vi "mod_Apply Doppler Filter.vi"(0 "input samples":cdb[](array[numeric]), 5 "doppler filter taps":dbl[](array[numeric]), 11 "error in (no error)":errorcluster, 13 "reset (T)":bool=TRUE) -> (4 "filtered output":cdb[](array[numeric]), 15 "error out":errorcluster)   [LabVIEW 2020, in "niDMT.lvlib"]
doc: "The input signal samples are filtered out through the Doppler filter, which is a kind of low-pass filter with the cut-off frequency of the Doppler frequency and with U-shaped passband gains, although other low-pass filters have flat or equi-ripple gains.\n\n\n Inputs:\n 1) Doppler frequency (Hz) \n - range : double precision\n 2) Input samples : the input signal samples in time domain\n 3) Sampling frequency : the sampling frequency of the input samples\n 4) Filter length : the number of taps in the filter\n\n Outputs:\n 1) Filtered output : the filtered output in time domain"
uses:
  <vilib>/addons/Modulation/niDMT.lvlib
  <vilib>/Analysis/3filter.llb/IIR Filter (DBL).vi
  <vilib>/Analysis/NI_AALBase.lvlib
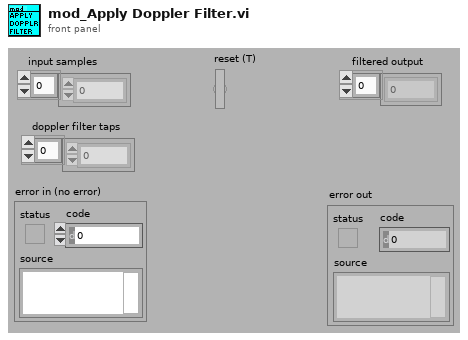
[diagram p1: front panel]
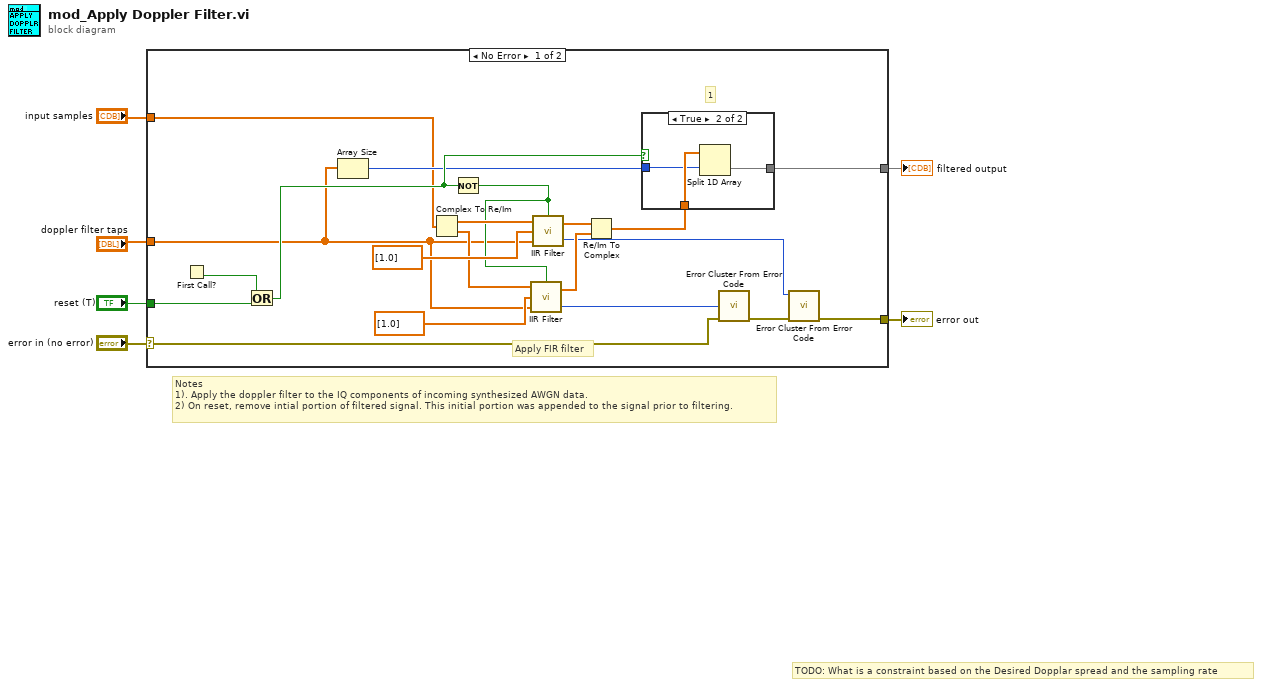
[diagram p0: block diagram]
diagram:
  # "Notes\n1). Apply the doppler filter to the IQ components of incoming synthesized AWGN data.\n2) On reset, remove intial portion of filtered signal. This initial portion was appended to the signal prior to filtering."
  # "TODO: What is a constraint based on the Desired Dopplar spread and the sampling rate"
  n1 = case shown="No Error" "error in (no error)" {
    selector: "error in (no error)" -> [w16 w31]
    tunnel: [w13 w31] -> w5
    tunnel: "input samples" -> [w10 _]
    tunnel: "doppler filter taps" -> [w9 _]
    tunnel: [w8 _] -> w2
    tunnel: "reset (T)" -> [w7 _]
    frame No Error {
      # "1"
      # "Apply FIR filter"
      n2 = First Call?() -> (First Call?: T/F=w26:bool)
      n3 = Or(x=w26, y=w7) -> (x .or. y?=w24:bool)
      n4 = Array Size(array=w9) -> (size(s)=w12:i32)
      n5 = Complex To Re/Im(x + iy=w10) -> (x=w23:dbl[], y=w22:dbl[])
      n6 = Not(x=w24) -> (.not. x?=w11:bool)
      n7 = call-poly <vilib>:"IIR Filter.vi"("init/cont (init:F)"=w11, "Forward Coefficients"=w9, "Reverse Coefficients"=dbl[] [1.0], "X"=w22) -> ("error"=w14:i32, "Filtered X"=w20:dbl[])
      n8 = call-poly <vilib>:"IIR Filter.vi"("init/cont (init:F)"=w11, "Forward Coefficients"=w9, "Reverse Coefficients"=dbl[] [1.0], "X"=w23) -> ("error"=w15:i32, "Filtered X"=w19:dbl[])
      n9 = Re/Im To Complex(1:w20, 2:w19) -> (0:w18:cdb[])
      n10 = case shown="True" w24 {
        tunnel: w18 -> [w27 w30]
        tunnel: [w27 w29] -> w8
        tunnel: w12 -> [_ w28]
        frame False {
        }
        frame True {
          n11 = Split 1D Array(array=w30, index=w28) -> (second subarray=w29:cdb[])  [unwired: 1 out]
        }
      }
      n12 = call <vilib>:"Error Cluster From Error Code.vi"("error in (no error)"=w16, "error code (0)"=w14) -> ("error out"=w17:errorcluster)  [unwired: 1 in, 6 out]
      n13 = call <vilib>:"Error Cluster From Error Code.vi"("error in (no error)"=w17, "error code (0)"=w15) -> ("error out"=w13:errorcluster)  [unwired: 1 in, 6 out]
    }
    frame Error {
    }
  }
  "error out" <- w5
  "filtered output" <- w2
